vi "Begin.vi"() -> (0 "error out":errorcluster)   [LabVIEW 2018]
doc: "Called before other user functions, this VI can be used to open I/O refnums, load in file data, and do general program initialization. Notice that the <B>error out</B> terminal is simply used for data flow. Wiring it to other structures or subVIs ensures that this VI runs first."
uses:
  <vilib>/Rock Robotics/WPI/DriverStation/WPI_DriverStationRobotMode2.ctl
  <vilib>/Rock Robotics/WPI/Joystick/WPI_JoystickDeviceEnum.ctl
  Odometry/Typedef/Odometry.ctl
  <vilib>/Rock Robotics/WPI/ThirdParty/REV Robotics/SPARK MAX/Typedef/Spark MAX Status Frames.ctl
  <vilib>/Rock Robotics/WPI/Solenoid/WPI_SolenoidChannel.ctl
  <vilib>/Rock Robotics/WPI/ThirdParty/REV Robotics/SPARK MAX/Typedef/Spark MAX Motor Type.ctl
  <vilib>/Rock Robotics/SystemInterfaces/DIO/FPGA_DIOChannel.ctl
  <vilib>/Rock Robotics/WPI/ThirdParty/REV Robotics/SPARK MAX/Typedef/Spark MAX Idle Mode.ctl
  Robot Global Data.vi
  <vilib>/Rock Robotics/Network Tables/NT Write String Array.vi
  <vilib>/Rock Robotics/WPI/Solenoid/WPI_SolenoidOpenDouble.vi
  <vilib>/Rock Robotics/WPI/Counter/WPI_CounterDigitalInputToDigitalSource.vi
  <vilib>/Rock Robotics/WPI/Counter/WPI_CounterOpen Semi Period Mode.vi
  <vilib>/Rock Robotics/SystemInterfaces/spilib/spi_bus.ctl
  Asynchronous TDMS Logger/TDMS Logger.lvclass
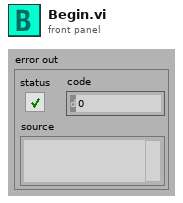
[diagram p1: front panel]
types:
  T1 = typedef "FPGA_DIOChannel.ctl" = enum8{"DIO 0", "DIO 1", "DIO 2", "DIO 3", "DIO 4", "DIO 5", "DIO 6", "DIO 7", "DIO 8", "DIO 9", "DIO MXP 0", "DIO MXP 1", "DIO MXP 2", "DIO MXP 3", "DIO MXP 4", "DIO MXP 5", "DIO MXP 6", "DIO MXP 7", "DIO MXP 8", "DIO MXP 9", "DIO MXP 10", "DIO MXP 11", "DIO MXP 12", "DIO MXP 13", "DIO MXP 14", "DIO MXP 15", "SPI Port CS1", "SPI Port CS2", "SPI Port CS3", "SPI Port MISO", "SPI Port MOSI", "Invalid"}
  T2 = typedef "Spark MAX Idle Mode.ctl" = enum16{"Coast", "Brake"}
  T3 = typedef "Spark MAX Motor Type.ctl" = enum16{"Brushed", "Brushless"}
  T4 = typedef "WPI_SolenoidChannel.ctl" = enum8{"Solenoid 0", "Solenoid 1", "Solenoid 2", "Solenoid 3", "Solenoid 4", "Solenoid 5", "Solenoid 6", "Solenoid 7", "Invalid"}
  T5 = typedef "Spark MAX Status Frames.ctl" = enum16{"Status 0", "Status 1", "Status 2"}
  T6 = cluster{"P Gain":dbl, "I Gain":dbl, "D Gain":dbl, "F Gain":dbl, "I Zone":dbl, "Min Output":dbl, "Max Output":dbl}
  T7 = typedef "WPI_JoystickDeviceEnum.ctl" = enum16{"USB 0", "USB 1", "USB 2", "USB 3", "USB 4", "USB 5"}
  T8 = typedef "Odometry.ctl" = cluster{"x":dbl, "y":dbl, "theta":dbl, "Left Encoder Raw":sgl, "Right Encoder Raw":sgl, "Left Velocity Raw":sgl, "Right Velocity Raw":sgl, "Left Encoder":dbl, "Right Encoder":dbl, "Late Iterations":i16}
  T9 = typedef "WPI_DriverStationRobotMode2.ctl" = enum16{"Autonomous Disabled", "Autonomous Enabled", "Teleop Disabled", "Teleop Enabled", "Disconnected", "Finish", "Test Disabled", "Test Enabled", "Emergency Stopped"}
  T10 = typedef "WPI_MotorControlDeviceRef.ctl" = cluster{"DeviceStatus":errorcluster, "Type":T11, "PWM":cluster{"PWM Channel":T12, "DeadBand":T13}, "CAN":cluster{"Device Number":u8, "SetOutput VI Ref":variant, "GetOutput VI Ref":variant, "Enable VI Ref":variant, "Disable VI Ref":variant, "Data":variant}, "Invert":bool, "DIO PWM":cluster{"PWM \"Enable\" Channel":T12, "DIOChannel":T1, "PWM Rate":dbl}}
  T11 = typedef "WPI_MotorControlType.ctl" = enum16{"PWM", "CAN", "DIO PWM"}
  T12 = typedef "FPGA_DIOPWMChannel.ctl" = enum8{"PWM 0", "PWM 1", "PWM 2", "PWM 3", "PWM 4", "PWM 5", "PWM 6", "PWM 7", "PWM 8", "PWM 9", "PWM MXP 0", "PWM MXP 1", "PWM MXP 2", "PWM MXP 3", "PWM MXP 4", "PWM MXP 5", "PWM MXP 6", "PWM MXP 7", "PWM MXP 8", "PWM MXP 9", "Invalid"}
  T13 = typedef "WPI_PWMDeadband.ctl" = cluster{"Name":string, "maxPositivePwm":i32, "minPositivePwm":i32, "centerPwm":i32, "maxNegativePwm":i32, "minNegativePwm":i32, "angularRange":u16}
  T14 = typedef "WPI_JoystickDevRef.ctl" = cluster{"Device":T7}
  T15 = typedef "spi_bus.ctl" = enum16{"SPI On-Board, CS0", "SPI On-Board, CS1", "SPI On-Board, CS2", "SPI On-Board, CS3", "SPI MXP", "Invalid"}
  T16 = typedef "WPI_GyroDevRef.ctl" = cluster{"DevStatus":errorcluster, "Analog Channel":T17, "Gain (VoltsPerDegree/Second)":dbl, "Gyro Type":enum16{"Analog", "XRS450"}, "Handle":i32, "SPI Bus":T15, "Device Found":bool, "Sample Rate":dbl, "Calibrate On Open":bool, "Offset":dbl}
  T17 = typedef "FPGA_AIChannel.ctl" = enum8{"AI 0", "AI 1", "AI 2", "AI 3", "AI MXP 0", "AI MXP 1", "AI MXP 2", "AI MXP 3", "Invalid"}
  T18 = typedef "SPARKMAX6Motor.ctl" = cluster{"FrontLeftMaster":T10, "FrontLeftSlave1":T10, "FrontLeftSlave2":T10, "FrontRightMaster":T10, "FrontRightSlave1":T10, "FrontRightSlave2":T10}
  T19 = typedef "WPI_DigitalInputDevRef.ctl" = cluster{"DevStatus":errorcluster, "DIO Channel":T1}
  T20 = typedef "FPGA_CounterEncoderSourceConvertionLVSourceType.ctl" = cluster{"DevStatus":errorcluster, "AnalogTriggerMode?":bool, "DigitalMode":cluster{"DIO Channel":T21}, "AnalogTriggerMode":cluster{"AnalogTriggerIndex":T22, "OutputType":T23}}
  T21 = typedef "FPGA_DIODigitalSourceChannel.ctl" = enum8{"DIO 0", "DIO 1", "DIO 2", "DIO 3", "DIO 4", "DIO 5", "DIO 6", "DIO 7", "DIO 8", "DIO 9", "DIO MXP 0", "DIO MXP 1", "DIO MXP 2", "DIO MXP 3", "DIO MXP 4", "DIO MXP 5", "DIO MXP 6", "DIO MXP 7", "DIO MXP 8", "DIO MXP 9", "DIO MXP 10", "DIO MXP 11", "DIO MXP 12", "DIO MXP 13", "DIO MXP 14", "DIO MXP 15", "SPI Port CS1", "SPI Port CS2", "SPI Port CS3", "SPI Port MISO", "SPI Port MOSI", "Disabled"}
  T22 = typedef "FPGA_AnalogTriggerIndex.ctl" = enum8{"Trig 0", "Trig 1", "Trig 2", "Trig 3", "Trig 4", "Trig 5", "Trig 6", "Trig 7", "Invalid"}
  T23 = typedef "FPGA_AnalogTriggerOutType.ctl" = enum16{"InWindow", "TriggerState", "Rising", "Falling"}
  T24 = typedef "WPI_CounterDevRef.ctl" = cluster{"DevStatus":errorcluster, "CntIndex":T25}
  T25 = typedef "FPGA_CounterCtrSystemIndex.ctl" = enum8{"Ctr 0", "Ctr 1", "Ctr 2", "Ctr 3", "Ctr 4", "Ctr 5", "Ctr 6", "Ctr 7", "Invalid"}
  T26 = typedef "WPI_SolenoidDevRef.ctl" = cluster{"DevStatus":errorcluster, "Pneumatics Control Module":u8, "Forward Solenoid Channel":T4, "Reverse Solenoid Channel":T4}
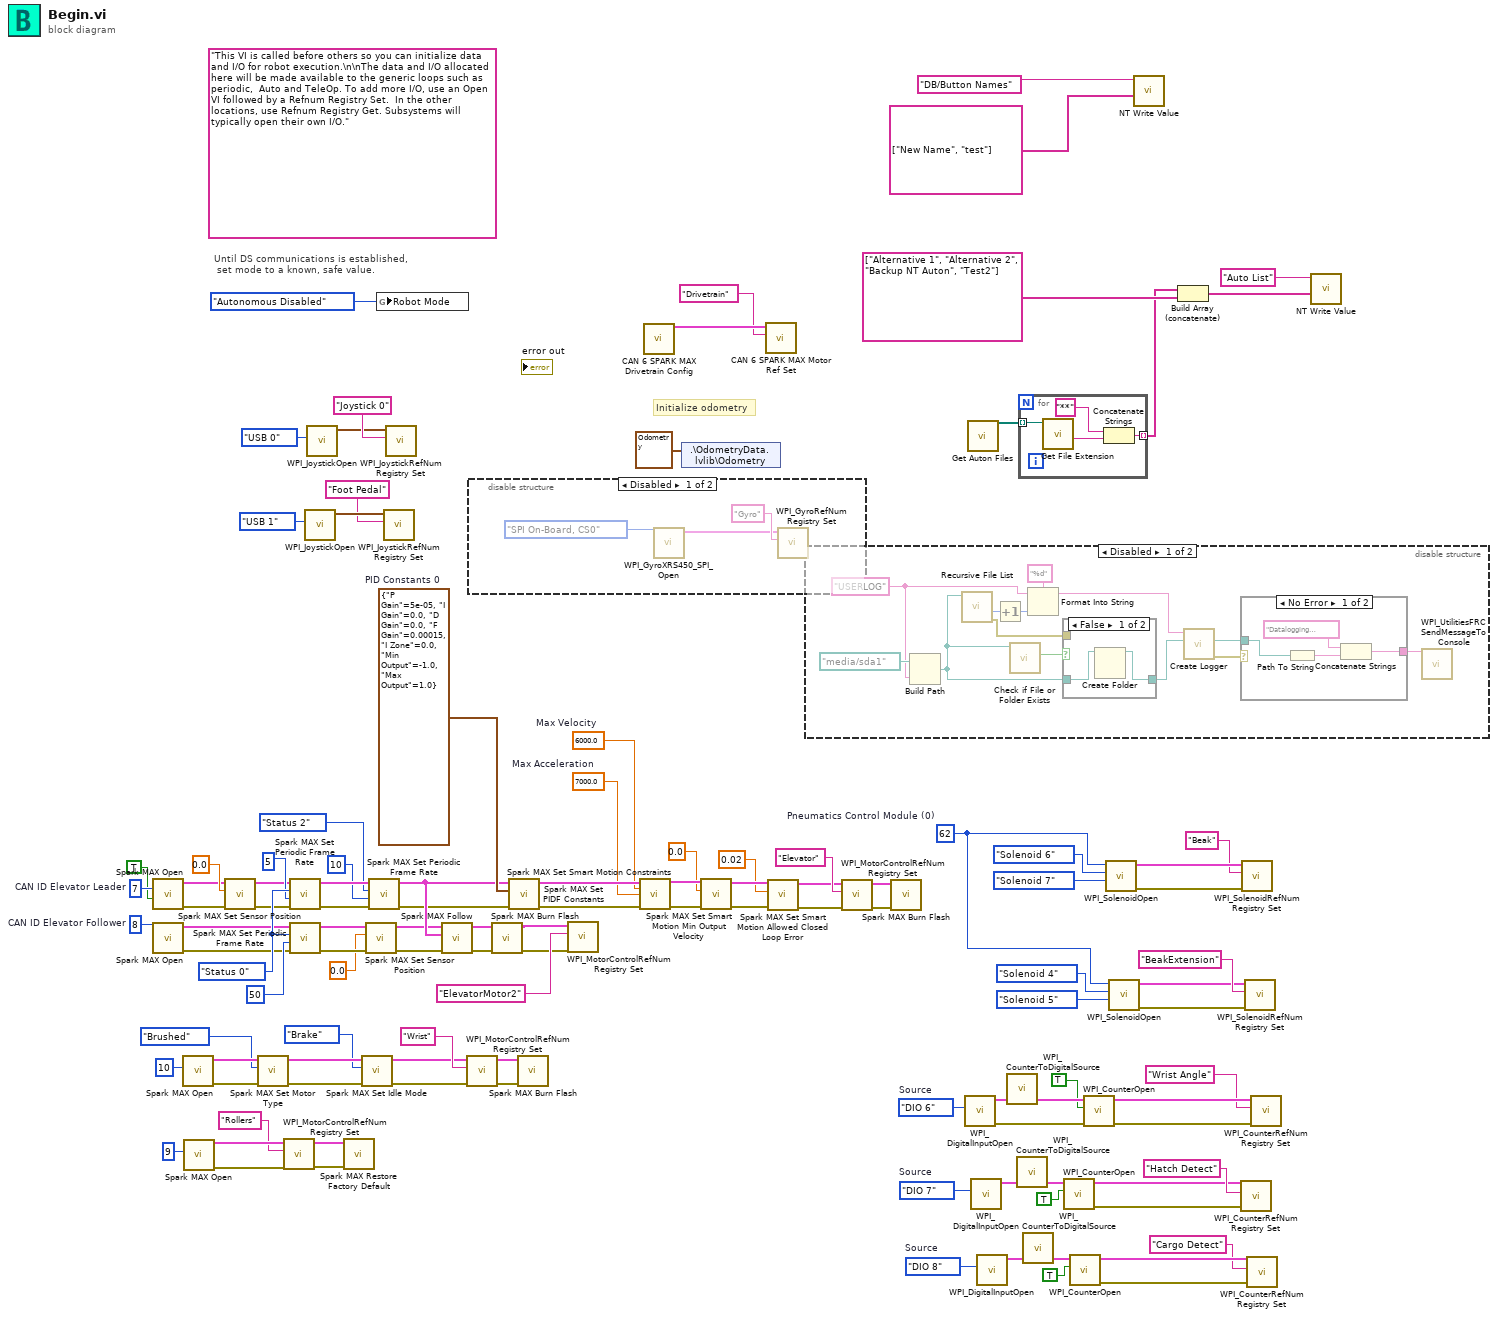
[diagram p0: block diagram]
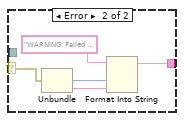
[diagram p3: hidden frame]
diagram:
  w2 = FPGA_DIOChannel."DIO 8"  # Source
  w21 = FPGA_DIOChannel."DIO 7"  # Source
  w37 = 7000.0  # Max Acceleration
  w38 = 6000.0  # Max Velocity
  w51 = FPGA_DIOChannel."DIO 6"  # Source
  w64 = u8 62  # Pneumatics Control Module (0)
  w95 = T6 {"P Gain"=5e-05, "I Gain"=0.0, "D Gain"=0.0, "F Gain"=0.00015, "I Zone"=0.0, "Min Output"=-1.0, "Max Output"=1.0}  # PID Constants 0
  w93 = Spark_MAX_Status_Frames."Status 0" ("Frame")
  w89 = u8 7  # CAN ID Elevator Leader
  w90 = u8 8  # CAN ID Elevator Follower
  (unwired) "This VI is called before others so you can initialize data and I/O for robot execution.\n\nThe data and I/O allocated here will be made available to the generic loops such as periodic,  Auto and TeleOp. To add more I/O, use an Open VI followed by a Refnum Registry Set.  In the other locations, use Refnum Registry Get. Subsystems will typically open their own I/O."
  # "Initialize odometry"
  # "Until DS communications is established,\n set mode to a known, safe value."
  n1 = call <vilib>:"Spark MAX Open.vi"("Invert"=TRUE, "Device Number"=w89) -> ("error out"=w79:errorcluster, "MotorControlDeviceRef"=w78:T10)  [unwired: 8 in]
  n2 = call <vilib>:"Spark MAX Open.vi"("Device Number"=w90) -> ("error out"=w91:errorcluster, "MotorControlDeviceRef"=w92:T10)  [unwired: 9 in]
  n3 = call <vilib>:"Spark MAX Open.vi"("Device Number"=u8 10) -> ("error out"=w32:errorcluster, "MotorControlDeviceRef"=w56:T10)  [unwired: 9 in]
  n4 = call <vilib>:"Spark MAX Open.vi"("Device Number"=u8 9) -> ("error out"=w25:errorcluster, "MotorControlDeviceRef"=w58:T10)  [unwired: 9 in]
  n5 = call <vilib>:"Spark MAX Set Sensor Position.vi"("error in"=w79, "Position"=0.0, "MotorControlDeviceRef"=w78) -> ("error out"=w76:errorcluster, "MotorControlDeviceRef"=w77:T10)  [unwired: 7 in]
  n6 = call <vilib>:"Spark MAX Set Motor Type.vi"("error in (no error)"=w32, "Enum"=Spark_MAX_Motor_Type."Brushed", "MotorControlDevRef"=w56) -> ("error out"=w53:errorcluster, "MotorControlDeviceRef"=w30:T10)  [unwired: 7 in]
  n7 = call <vilib>:"WPI_MotorControlRefNum Registry Set.vi"("error in (no error)"=w25, "refnum name"="Rollers", "MotorControlDevRef"=w58) -> ("error out"=w24:errorcluster, "MotorControlDevRef"=w23:T10)  [unwired: 7 in]
  n8 = call <vilib>:"Spark MAX Set Periodic Frame Rate.vi"("error in"=w76, "Frame rate (ms)"=u16 5, "Frame"=w93, "MotorControlDeviceRef"=w77) -> ("error out"=w88:errorcluster, "MotorControlDeviceRef"=w87:T10)  [unwired: 6 in]
  n9 = call <vilib>:"Spark MAX Set Periodic Frame Rate.vi"("error in"=w91, "Frame rate (ms)"=u16 50, "Frame"=w93, "MotorControlDeviceRef"=w92) -> ("error out"=w11:errorcluster, "MotorControlDeviceRef"=w12:T10)  [unwired: 6 in]
  n10 = call <vilib>:"WPI_JoystickOpen.vi"("JoystickDevice"=WPI_JoystickDeviceEnum."USB 1") -> ("JoystickDevRef"=w105:T14)  [unwired: 10 in]
  n11 = call <vilib>:"WPI_JoystickOpen.vi"("JoystickDevice"=WPI_JoystickDeviceEnum."USB 0") -> ("JoystickDevRef"=w111:T14)  [unwired: 10 in]
  n12 = call <vilib>:"Spark MAX Restore Factory Default.vi"("error in"=w24, "MotorControlDeviceRef"=w23) -> ()  [unwired: 8 in, 2 out]
  n13 = call <vilib>:"Spark MAX Set Idle Mode.vi"("error in (no error)"=w53, "Idle Mode"=Spark_MAX_Idle_Mode."Brake", "MotorControlDeviceRef in"=w30) -> ("error out"=w31:errorcluster, "MotorControlDeviceRef out"=w29:T10)  [unwired: 7 in]
  n14 = call <vilib>:"Spark MAX Set Sensor Position.vi"("error in"=w11, "Position"=0.0, "MotorControlDeviceRef"=w12) -> ("error out"=w9:errorcluster, "MotorControlDeviceRef"=w10:T10)  [unwired: 7 in]
  n15 = call <vilib>:"Spark MAX Set Periodic Frame Rate.vi"("error in"=w88, "Frame rate (ms)"=u16 10, "Frame"=Spark_MAX_Status_Frames."Status 2", "MotorControlDeviceRef"=w87) -> ("error out"=w84:errorcluster, "MotorControlDeviceRef"=w86:T10)  [unwired: 6 in]
  n16 = global write "Robot Global Data.vi" "Robot Mode"(WPI_DriverStationRobotMode2."Autonomous Disabled" ("Robot Mode")) -> ()
  n17 = call <vilib>:"WPI_JoystickRefNum Registry Set.vi"("refnum name"="Foot Pedal", "JoystickDevRef"=w105) -> ()  [unwired: 8 in, 2 out]
  n18 = call <vilib>:"WPI_JoystickRefNum Registry Set.vi"("refnum name"="Joystick 0", "JoystickDevRef"=w111) -> ()  [unwired: 8 in, 2 out]
  n19 = call <vilib>:"Spark MAX Follow.vi"("error in (no error)"=w9, "Master Controller"=w86, "MotorControlDeviceRef"=w10) -> ("error out"=w62:errorcluster, "MotorControlDeviceRef"=w61:T10)  [unwired: 7 in]
  n20 = call <vilib>:"WPI_MotorControlRefNum Registry Set.vi"("error in (no error)"=w31, "refnum name"="Wrist", "MotorControlDevRef"=w29) -> ("error out"=w27:errorcluster, "MotorControlDevRef"=w26:T10)  [unwired: 7 in]
  n21 = disable-structure shown="Disabled" {
    frame Disabled {
      n22 = call <vilib>:"WPI_GyroXRS450_SPI_Open.vi"("SPI Bus"=spi_bus."SPI On-Board, CS0") -> ("GyroDevRef"=w114:T16)  [unwired: 8 in, 2 out]
      n23 = call <vilib>:"WPI_GyroRefNum Registry Set.vi"("refnum name"="Gyro", "GyroDevRef"=w114) -> ()  [unwired: 8 in, 2 out]
    }
    frame Enabled {
    }
  }
  n24 = call <vilib>:"Spark MAX Burn Flash.vi"("error in"=w62, "MotorControlDeviceRef"=w61) -> ("error out"=w14:errorcluster, "MotorControlDeviceRef"=w13:T10)  [unwired: 8 in]
  n25 = call <vilib>:"Spark MAX Set PIDF Constants.vi"("error in"=w84, "PID Constants"=w95, "MotorControlDeviceRef"=w86) -> ("error out"=w82:errorcluster, "MotorControlDeviceRef"=w81:T10)  [unwired: 7 in]
  n26 = call <vilib>:"Spark MAX Burn Flash.vi"("error in"=w27, "MotorControlDeviceRef"=w26) -> ()  [unwired: 8 in, 2 out]
  n27 = call <vilib>:"WPI_MotorControlRefNum Registry Set.vi"("error in (no error)"=w14, "refnum name"="ElevatorMotor2", "MotorControlDevRef"=w13) -> ()  [unwired: 7 in, 2 out]
  n28 = call <vilib>:"Spark MAX Set Smart Motion Constraints.vi"("MotorControlDeviceRef"=w81, "Max Velocity"=w38, "Max Acceleration"=w37, "error in"=w82) -> ("MotorControlDeviceRef"=w43:T10, "error out"=w44:errorcluster)  [unwired: 10 in]
  n29 = call "CAN 6 SPARK MAX Drivetrain Config.vi"() -> ("SPARK MAX Ref"=w98:T18)  [unwired: 19 in]
  n30 = shared-variable ".\\OdometryData.lvlib\\Odometry"(T8 {"x"=0.0, "y"=0.0, "theta"=0.0, "Left Encoder Raw"=0.0, "Right Encoder Raw"=0.0, "Left Velocity Raw"=0.0, "Right Velocity Raw"=0.0, "Left Encoder"=0.0, "Right Encoder"=0.0, "Late Iterations"=0} ("Odometry")) -> ()  [unwired: 1 in, 1 out]
  n31 = call <vilib>:"Spark MAX Set Smart Motion Min Output Velocity.vi"("error in"=w44, "Minimum Velocity Output"=0.0, "MotorControlDeviceRef"=w43) -> ("error out"=w42:errorcluster, "MotorControlDeviceRef"=w41:T10)  [unwired: 7 in]
  n32 = call "CAN 6 SPARK MAX Motor Ref Set.vi"("refnum name"="Drivetrain", "TalonSRX6MotorRef in"=w98) -> ()  [unwired: 8 in, 2 out]
  n33 = call <vilib>:"Spark MAX Set Smart Motion Allowed Closed Loop Error.vi"("error in"=w42, "Allowed Closed Loop Error"=0.02, "MotorControlDeviceRef"=w41) -> ("error out"=w40:errorcluster, "MotorControlDeviceRef"=w39:T10)  [unwired: 7 in]
  n34 = disable-structure shown="Disabled" {
    frame Disabled {
      w124 = "USERLOG" ("Base File Name")
      n35 = Build Path(base path=path "/media/sda1", name or relative path=w124) -> (appended path=w126:path)
      n36 = call <vilib>:"Recursive File List.vi"("Folder Path"=w126) -> ("error out"=w121:errorcluster, "Number of Files"=w125:i32)  [unwired: 6 in, 3 out]
      n37 = Increment(x=w125) -> (x+1=w123:i32)
      n38 = call <vilib>:"Check if File or Folder Exists.vi"("path"=w126) -> ("file or folder exists?"=w127:bool)  [unwired: 8 in, 2 out]
      n39 = Format Into String(format string="%d", initial string=w124, w123) -> (resulting string=w120:string)  [unwired: 1 in, 1 out]
      n40 = case shown="False" w127 {
        tunnel: w126 -> [w131 w132]
        tunnel: [w130 w132] -> w117
        tunnel: w121 -> [_ _]
        frame False {
          n41 = Create Folder(path (use dialog)=w131) -> (created path=w130:path)  [unwired: 2 in, 2 out]
        }
        frame True {
        }
      }
      n42 = call "Create Logger.vi"("Base Folder"=w117, "Base File Name"=w120) -> ("Error Out"=w118:errorcluster, "Final Path"=w119:path)  [unwired: 7 in, 1 out]
      n43 = case shown="No Error" w118 {
        selector: w118 -> [_ w140]
        tunnel: w119 -> [w136 _]
        tunnel: [w133 w137] -> w129
        frame No Error {
          n44 = Path To String(path=w136) -> (string=w135:string)
          n45 = Concatenate Strings("Datalogging Initialized to: " ("string"), w135) -> (w133:string)
        }
        frame Error {
          n46 = Unbundle(w140) -> ("code"=w139:i32, "source"=w138:string)  [unwired: 1 out]
          n47 = Format Into String(initial string="WARNING: Failed to initialize datalogger! " ("string"), w139, w138) -> (resulting string=w137:string)  [unwired: 2 in, 1 out]
        }
      }
      n48 = call <vilib>:"WPI_UtilitiesFRC SendMessageToConsole.vi"("Message"=w129) -> ()  [unwired: 14 in, 1 out]
    }
    frame Enabled {
    }
  }
  n49 = call <vilib>:"WPI_MotorControlRefNum Registry Set.vi"("error in (no error)"=w40, "refnum name"="Elevator", "MotorControlDevRef"=w39) -> ("error out"=w33:errorcluster, "MotorControlDevRef"=w34:T10)  [unwired: 7 in]
  n50 = call <vilib>:"Spark MAX Burn Flash.vi"("error in"=w33, "MotorControlDeviceRef"=w34) -> ()  [unwired: 8 in, 2 out]
  n51 = call <vilib>:"WPI_DigitalInputOpen.vi"("DIO Channel"=w51) -> ("error out"=w49:errorcluster, "DigitalInputDevRef"=w50:T19)  [unwired: 1 in, 8 out]
  n52 = call "Get Auton Files.vi"() -> ("All Files in Dir"=w101:path[])  [unwired: 11 in]
  n53 = call <vilib>:"WPI_DigitalInputOpen.vi"("DIO Channel"=w21) -> ("DigitalInputDevRef"=w20:T19)  [unwired: 1 in, 9 out]
  n54 = call <vilib>:"WPI_DigitalInputOpen.vi"("DIO Channel"=w2) -> ("DigitalInputDevRef"=w3:T19)  [unwired: 1 in, 9 out]
  n55 = call-poly <vilib>:"WPI_CounterToDigitalSource.vi"("DigitalInputDevRef"=w50) -> ("Digital Source"=w52:T20)  [unwired: 6 out]
  n56 = call-poly <vilib>:"WPI_CounterToDigitalSource.vi"("DigitalInputDevRef"=w20) -> ("Digital Source"=w22:T20)  [unwired: 6 out]
  n57 = for {
    tunnel: w101 -> [w145] mode=indexing
    tunnel: [w142] -> w100 mode=indexing
    n58 = call <vilib>:"Get File Extension.vi"("file"=w145) -> ("filename without extension"=w144:string)  [unwired: 6 in, 4 out]
    n59 = Concatenate Strings("**" ("string"), w144) -> (w142:string)
  }
  n60 = call-poly <vilib>:"WPI_CounterToDigitalSource.vi"("DigitalInputDevRef"=w3) -> ("Digital Source"=w1:T20)  [unwired: 6 out]
  n61 = call-poly <vilib>:"WPI_CounterOpen.vi"("High Pulse (T)"=TRUE, "Source"=w22) -> ("error out"=w16:errorcluster, "CounterDevRef"=w17:T24)  [unwired: 3 in, 5 out]
  n62 = call-poly <vilib>:"WPI_CounterOpen.vi"("High Pulse (T)"=TRUE, "Source"=w1) -> ("error out"=w7:errorcluster, "CounterDevRef"=w6:T24)  [unwired: 3 in, 5 out]
  n63 = call-poly <vilib>:"WPI_CounterOpen.vi"("error in (no error)"=w49, "High Pulse (T)"=TRUE, "Source"=w52) -> ("error out"=w47:errorcluster, "CounterDevRef"=w48:T24)  [unwired: 2 in, 5 out]
  n64 = call-poly <vilib>:"WPI_SolenoidOpen.vi"("Reverse Solenoid Channel"=WPI_SolenoidChannel."Solenoid 7", "Forward Solenoid Channel"=WPI_SolenoidChannel."Solenoid 6", "Pneumatics Control Module (0)"=w64) -> ("error out"=w73:errorcluster, "SolenoidDevRef"=w74:T26)  [unwired: 7 in]
  n65 = call-poly <vilib>:"WPI_SolenoidOpen.vi"("Reverse Solenoid Channel"=WPI_SolenoidChannel."Solenoid 5", "Forward Solenoid Channel"=WPI_SolenoidChannel."Solenoid 4", "Pneumatics Control Module (0)"=w64) -> ("error out"=w66:errorcluster, "SolenoidDevRef"=w65:T26)  [unwired: 7 in]
  n66 = call-poly <vilib>:"NT Write Value.vi"("String Array"=string[] ["New Name", "test"], "Name"="DB/Button Names") -> ()  [unwired: 9 in, 1 out]
  n67 = Build Array (concatenate)(w100, string[] ["Alternative 1", "Alternative 2", "Backup NT Auton", "Test2"] ("String Array")) -> (w99:string[])
  n68 = call <vilib>:"WPI_CounterRefNum Registry Set.vi"("error in (no error)"=w16, "refnum name"="Hatch Detect", "CounterDevRef"=w17) -> ()  [unwired: 7 in, 2 out]
  n69 = call <vilib>:"WPI_SolenoidRefNum Registry Set.vi"("error in (no error)"=w73, "refnum name"="Beak", "SolenoidDevRef"=w74) -> ()  [unwired: 7 in, 2 out]
  n70 = call <vilib>:"WPI_SolenoidRefNum Registry Set.vi"("error in (no error)"=w66, "refnum name"="BeakExtension", "SolenoidDevRef"=w65) -> ()  [unwired: 7 in, 2 out]
  n71 = call <vilib>:"WPI_CounterRefNum Registry Set.vi"("error in (no error)"=w7, "refnum name"="Cargo Detect", "CounterDevRef"=w6) -> ()  [unwired: 7 in, 2 out]
  n72 = call <vilib>:"WPI_CounterRefNum Registry Set.vi"("error in (no error)"=w47, "refnum name"="Wrist Angle", "CounterDevRef"=w48) -> ()  [unwired: 7 in, 2 out]
  n73 = call-poly <vilib>:"NT Write Value.vi"("String Array"=w99, "Name"="Auto List") -> ()  [unwired: 9 in, 1 out]
